vi "State Machine.vi"() -> ()   [LabVIEW 2010]
doc: "이 VI는 상태 머신의 템플릿입니다. 더 많은 프로세스를 추가하려면, 타입 정의된 열거형 상수를 수정합니다. 열거형 순서는 클러스터 순서와 일치해야 합니다."
uses:
  State Enum.ctl
panel:
  in  "메뉴":T1
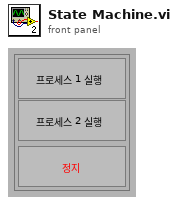
[diagram p1: front panel]
types:
  T1 = cluster{"Process 1":bool, "Process 2":bool, "stop":bool}
  T2 = typedef "State Enum.ctl" = enum32{"유휴", "프로세스 1", "프로세스 2", "정지"}
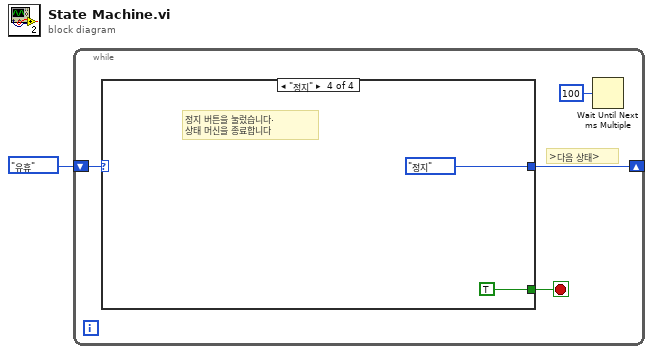
[diagram p0: block diagram]
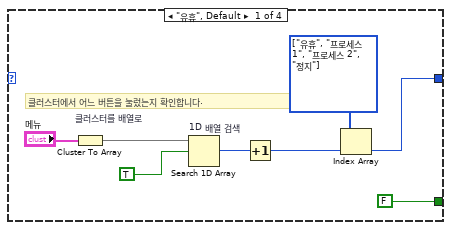
[diagram p2: hidden frame]
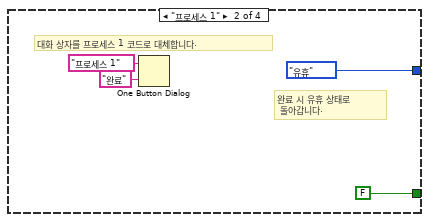
[diagram p3: hidden frame]
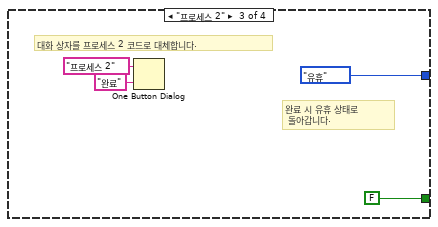
[diagram p4: hidden frame]
diagram:
  n1 = while {
    shift-right: [w4] -> _
    shift-left: State_Enum."유휴" ("Enum") -> [w5]
    stop <- w3 stop-if-true
    # ">다음 상태>"
    n2 = case shown="\"정지\"" w5 {
      tunnel: [w6 State_Enum."유휴" ("Enum") State_Enum."유휴" ("Enum") State_Enum."정지" ("Enum")] -> w4
      tunnel: [FALSE FALSE FALSE TRUE] -> w3
      frame "유휴", Default {
        w7 = T2[] [enum."유휴", enum."프로세스 1", enum."프로세스 2", enum."정지"] items=["유휴", "프로세스 1", "프로세스 2", "정지"]
        # "클러스터에서 어느 버튼을 눌렀는지 확인합니다."
        n3 = Cluster To Array "클러스터를 배열로"(cluster="메뉴") -> (array=w12:bool[])
        n4 = Search 1D Array "1D 배열 검색"(1D array=w12, element=TRUE) -> (index of element=w9:i32)  [unwired: 1 in]
        n5 = Increment(x=w9) -> (x+1=w8:i32)
        n6 = Index Array(array=w7, index=w8) -> (element=w6:T2)
      }
      frame "프로세스 1" {
        # "완료 시 유휴 상태로\n 돌아갑니다."
        # "대화 상자를 프로세스 1 코드로 대체합니다."
        n7 = One Button Dialog(message="프로세스 1", button name ("OK")="완료") -> ()  [unwired: 1 out]
      }
      frame "프로세스 2" {
        # "대화 상자를 프로세스 2 코드로 대체합니다."
        # "완료 시 유휴 상태로\n 돌아갑니다."
        n8 = One Button Dialog(message="프로세스 2", button name ("OK")="완료") -> ()  [unwired: 1 out]
      }
      frame "정지" {
        # "정지 버튼을 눌렀습니다.\n상태 머신을 종료합니다"
      }
    }
    n9 = Wait Until Next ms Multiple(millisecond multiple=u32 100) -> ()  [unwired: 1 out]
  }
